vi "instrumentProperties_series.vi"(5 "error in (no error)":errorcluster, 7 "specIndex":u16) -> (15 "OSA series":T1, 19 "error out":errorcluster)   [LabVIEW 2010, in "OSA.lvclass"]
doc: "Gets the OSA series, (OSA200 or OSA300)."
uses:
  OSA.lvclass
  typeDef/OSA_series.ctl
  FTSLib.dll
  OSA20X_misc.lvlib
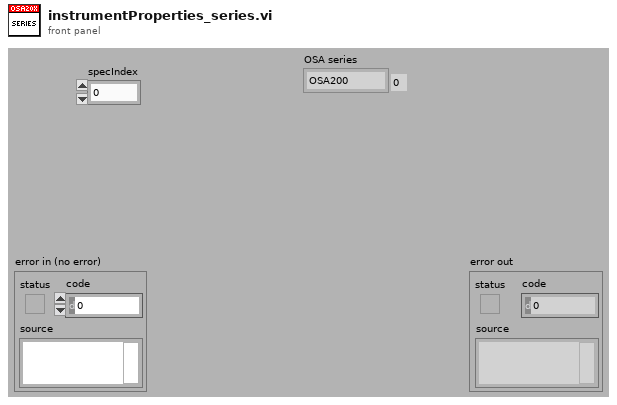
[diagram p1: front panel]
types:
  T1 = typedef "OSA.lvclass/OSA_series.ctl" = enum16{"OSA200", "OSA300", "UNKNOWN"}
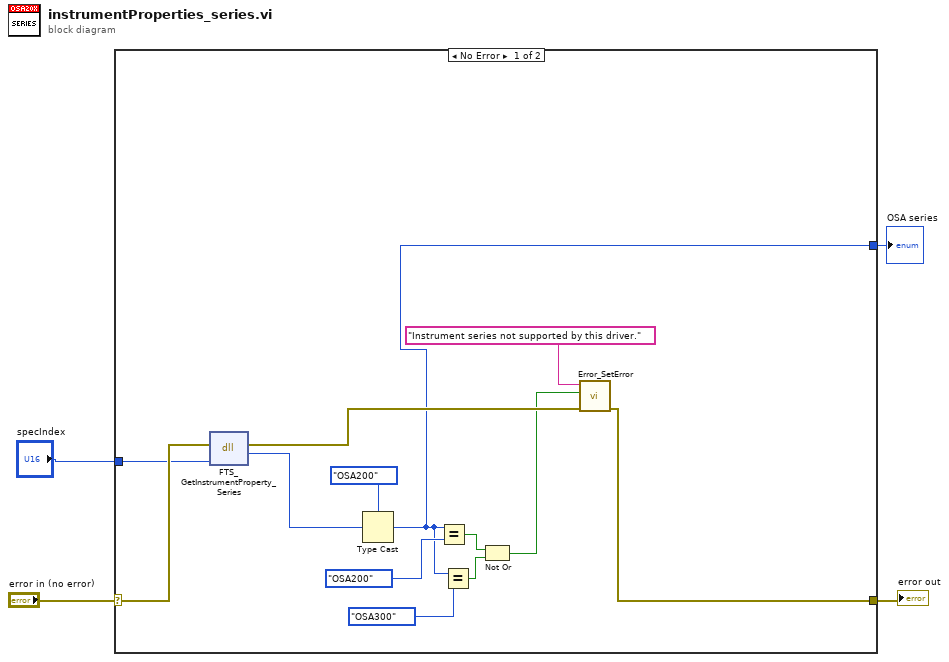
[diagram p0: block diagram]
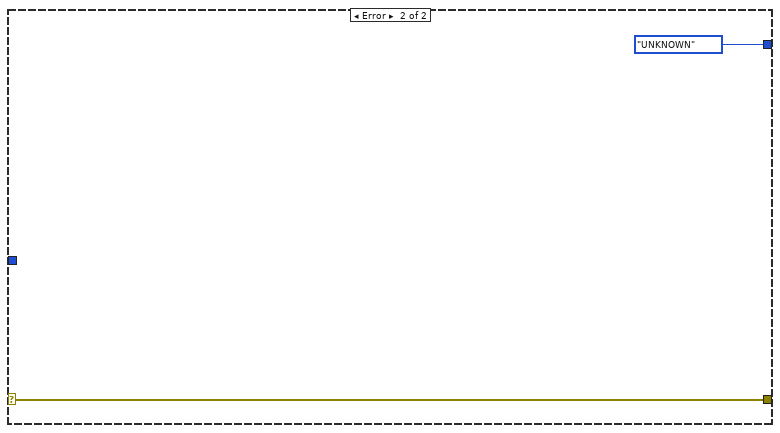
[diagram p2: hidden frame]
diagram:
  n1 = case shown="No Error" "error in (no error)" {
    selector: "error in (no error)" -> [w17 w19]
    tunnel: [w6 w19] -> w3
    tunnel: "specIndex" -> [w16 _]
    tunnel: [w5 OSA_series."UNKNOWN" ("OSA series")] -> w1
    frame No Error {
      n2 = dll-call lib="FTSLib.*" fn="FTS_GetInstrumentProperty_Series"(error in=w17, "specIndex"=w16) -> (error out=w15:errorcluster, "return type"=w14:u16)  [unwired: 3 in, 1 out]
      n3 = Type Cast(type=OSA_series."OSA200" ("OSA series"), x=w14) -> (*(type *) &x=w5:T1)
      n4 = Equal?(x=w5, y=OSA_series."OSA200") -> (x = y?=w10:bool)
      n5 = Equal?(x=w5, y=OSA_series."OSA300") -> (x = y?=w9:bool)
      n6 = Not Or(1:w9, 2:w10) -> (0:w8:bool)
      n7 = call "Error_SetError.vi"("error in"=w15, "status (true)"=w8, "source(\"\")"="Instrument series not supported by this driver." ("source(\"\")")) -> ("error out"=w6:errorcluster)  [unwired: 4 in]
    }
    frame Error {
    }
  }
  "error out" <- w3
  "OSA series" <- w1
